vi "Decimate.vi"(1 "increment":i32=3, 2 "array":i32[](array[numeric])) -> (0 "decimated array":i32[](array[numeric]))   [LabVIEW 2021]
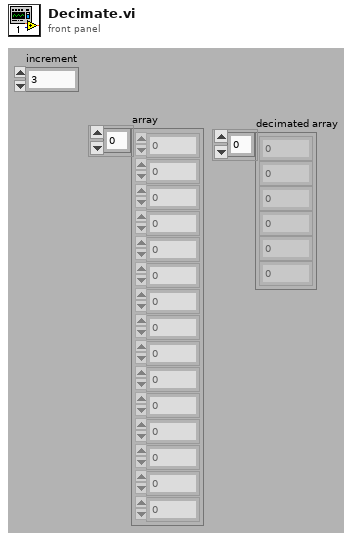
[diagram p1: front panel]
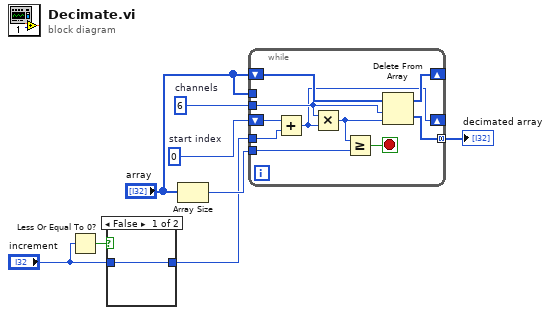
[diagram p0: block diagram]
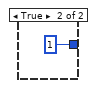
[diagram p2: hidden frame]
diagram:
  w4 = 6  # channels
  w8 = 0  # start index
  n1 = Less Or Equal To 0?(x="increment") -> (x <= 0?=w3:bool)
  n2 = case shown="False" w3 {
    tunnel: "increment" -> [w9 _]
    tunnel: [w9 1] -> w1
    frame False {
    }
    frame True {
    }
  }
  n3 = Array Size(array="array") -> (size(s)=w7:i32)
  n4 = while {
    tunnel: "array" -> [_]
    shift-right: [w13] -> _
    shift-left: w8 -> [w20]
    tunnel: w1 -> [w19]
    tunnel: w7 -> [w18]
    shift-right: [w15] -> _
    shift-left: "array" -> [w16]
    tunnel: w4 -> [w14]
    tunnel: [w12] -> w5 mode=concatenating
    stop <- w17 stop-if-true
    n5 = Add(x=w20, y=w19) -> (x+y=w13:i32)
    n6 = Multiply(x=w14, y=w13) -> (x*y=w11:i32)
    n7 = Greater Or Equal?(x=w11, y=w18) -> (x >= y?=w17:bool)
    n8 = Delete From Array(array=w16, length=w14, index=w11) -> (deleted portion=w12:i32[], array with subset deleted=w15:i32[])
  }
  "decimated array" <- w5
